vi "Search for Attribute.vi"(8 "error in (no error)":errorcluster, 10 "package attribute name":string, 11 "package attributes CLI string in":string) -> (0 "error out":errorcluster, 1 "string after attribute":string, 2 "string matching attribute":string, 3 "string before attribute":string, 4 "package attribute string":string, 5 "attribute found?":bool)   [LabVIEW 2014, in "NIPM_API.lvlib"]
doc: "This VI searches for the first match of a package attribute in a package attributes string.\n\nINPUT(s)\n<B>Package attributes CLI string</B>: This is a string containing the package attributes. This string can come from certain nipkg CLI commands as well as the control file text.\n\n<B>Package attribute name</B>: This is the name of the package attribute.\n\nOUTPUT(s)\n<B>String before attribute</B>: This returns the substring before the package attribute string. If the package attribute is not found, then this returns an empty string.\n\n<B>String matching attribute</B>: This returns the matching substring for the package attribute (e.g. \"Maintainer: \". If the package attribute is not found, then this returns an empty string.\n\n<B>String after attribute</B>: This returns the substring after the first matching package attribute string. If the package attribute is not found, then this returns an empty string.\n\n<B>Attribute found?</B>: Returns if the package attribute is found in the package attribute string. Note: If the package attribute is an empty string, this output will return a FALSE.\n\n<B>Package attribute string</B>: This output contains the package attribute string containing the colon and space (e.g. \"Package: \", \"Depends: \", \"Maintainer: \", etc), even if the package attribute is not found."
uses:
  NIPM_API.lvlib
  <vilib>/regexp/Match Regular Expression.xnode
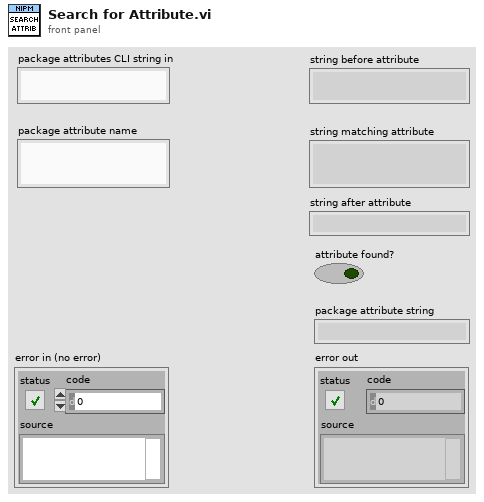
[diagram p1: front panel]
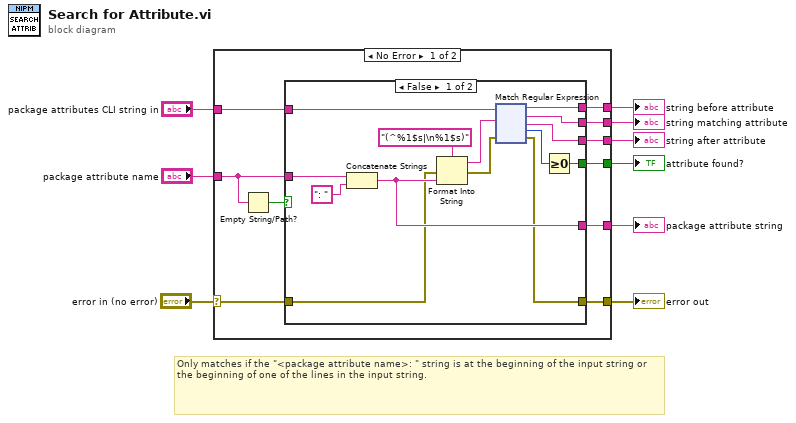
[diagram p0: block diagram]
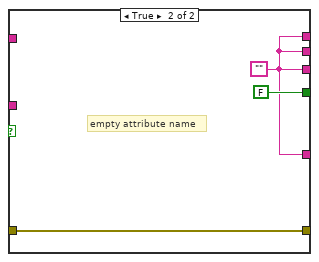
[diagram p2: hidden frame]
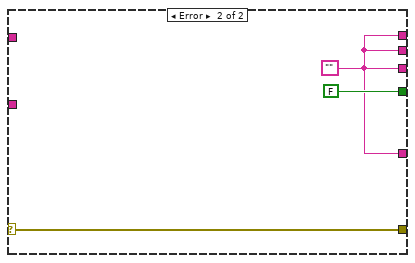
[diagram p3: hidden frame]
diagram:
  # "Only matches if the \"<package attribute name>: \" string is at the beginning of the input string or the beginning of one of the lines in the input string."
  n1 = case shown="No Error" "error in (no error)" {
    selector: "error in (no error)" -> [w11 w153]
    tunnel: [w18 FALSE] -> w9
    tunnel: "package attribute name" -> [w17 _]
    tunnel: "package attributes CLI string in" -> [w16 _]
    tunnel: [w15 w151] -> w6
    tunnel: [w10 w153] -> w4
    tunnel: [w14 w151] -> w2
    tunnel: [w13 w151] -> w3
    tunnel: [w12 w151] -> w1
    frame No Error {
      n2 = Empty String/Path?(string/path=w17) -> (empty?=w19:bool)
      n3 = case shown="False" w19 {
        tunnel: [w33 w149] -> w15
        tunnel: w16 -> [w24 _]
        tunnel: w17 -> [w31 _]
        tunnel: [w30 FALSE] -> w18
        tunnel: [w29 w149] -> w13
        tunnel: [w28 w149] -> w14
        tunnel: [w26 w149] -> w12
        tunnel: w11 -> [w22 w148]
        tunnel: [w20 w148] -> w10
        frame False {
          n4 = Concatenate Strings(w31, ": " ("string")) -> (w26:string)
          n5 = Format Into String(format string="(^%1$s|\n%1$s)", error in=w22, w26) -> (resulting string=w25:string, error out=w21:errorcluster)  [unwired: 1 in]
          n6 = xnode "Match Regular Expression"("input string"=w24, "regular expression"=w25, "error in"=w21) -> ("before match"=w29:string, "whole match"=w28:string, "after match"=w33:string, "offset past match"=w23:i32, "error out"=w20:errorcluster)  [unwired: 3 in]
          n7 = Greater Or Equal To 0?(x=w23) -> (x >= 0?=w30:bool)
        }
        frame True {
          w149 = ""
          # "empty attribute name"
        }
      }
    }
    frame Error {
      w151 = ""
    }
  }
  "attribute found?" <- w9
  "string after attribute" <- w6
  "error out" <- w4
  "string before attribute" <- w3
  "string matching attribute" <- w2
  "package attribute string" <- w1
